vi "WOBOT 2020 Vision.vi"() -> ()   [LabVIEW 2025]
uses:
  Ctrls/Battery Control.ctl
  <vilib>/Utility/sysdir.llb/System Directory Type.ctl
  Camera Set Up/Event/Event Setup Types.ctl
  <vilib>/vision/Image Controls.llb/IMAQ Image.ctl
  <vilib>/Utility/config.llb/Read Key (String).vi
  <vilib>/Utility/config.llb/Write Key (String).vi
  <vilib>/Rock Robotics/Network Tables/NT Read Boolean.vi
  <vilib>/Rock Robotics/Network Tables/NT Read String.vi
  <vilib>/Rock Robotics/Network Tables/NT Write Boolean.vi
  <vilib>/Utility/config.llb/NI_LVConfig.lvlib
panel:
  in  "Tab Control":enum32{"Post Processed", "Post Processed 2"}(tab)
  in  "Exit":bool
  out "DS Talking":bool
  out "NT Table":bool
  out "Title":string="Wobot 2020 Vision Ver 1.0.6"
  in  "Save":bool
  out "Vision Computer IP Address":string="DESKTOP-BLQQPIQ"
  out "Attached Cameras":string[](array[string])
  out "Rio Talking":bool
  in  "TEAM":u32=141
  out "Vision Battery Power (%)":T1 scale=0.0..100.0
  out "Driver Station IP":string
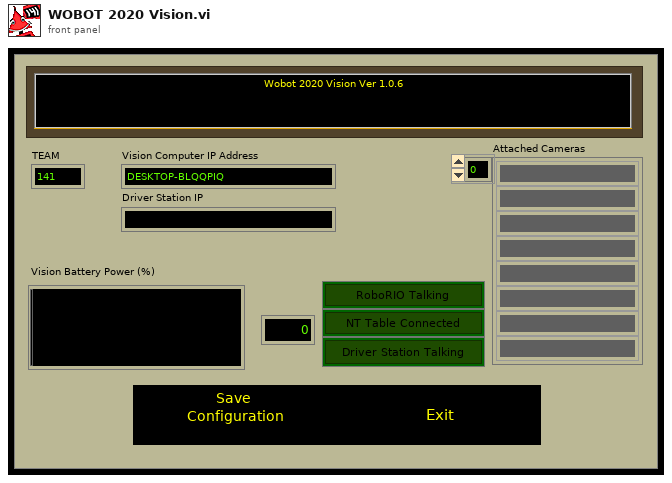
[diagram p1: front panel]
types:
  T1 = typedef "Battery Control.ctl" = u8
  T2 = typedef "System Directory Type.ctl" = i32
  T3 = typedef "Event Setup Types.ctl" = enum16{"Default", "Camera Loop Started", "GreyScale", "Reset Camera Settings", "Reset Team Number", "Save Data", "Setting Changed", "Update Video Mode", "Video Mode Changed", "Exit"}
  T4 = typedef "NI_LVConfig.lvlib/Config Data RefNum.ctl" = refnum<k1>
  T5 = typedef "IMAQ Image.ctl" = refnum<image>
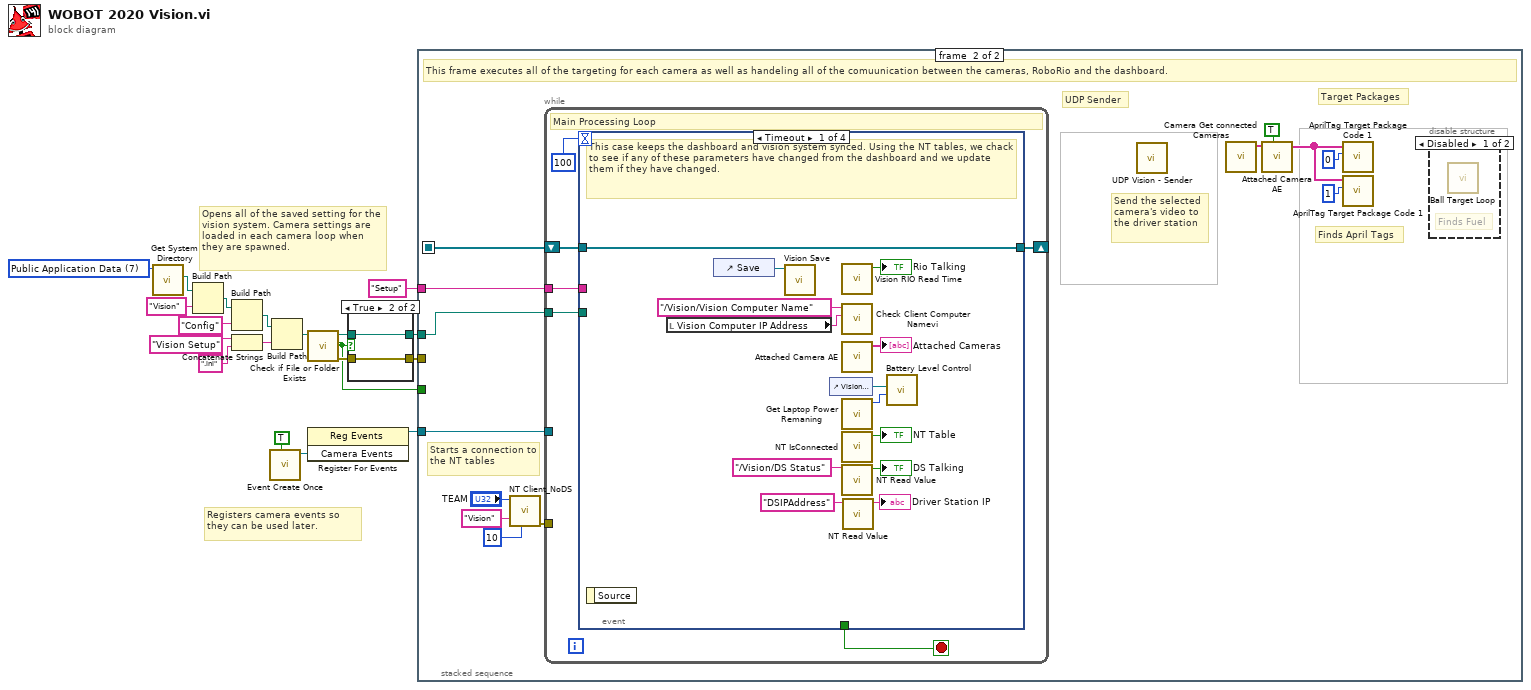
[diagram p0: block diagram]
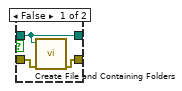
[diagram p2: hidden frame]
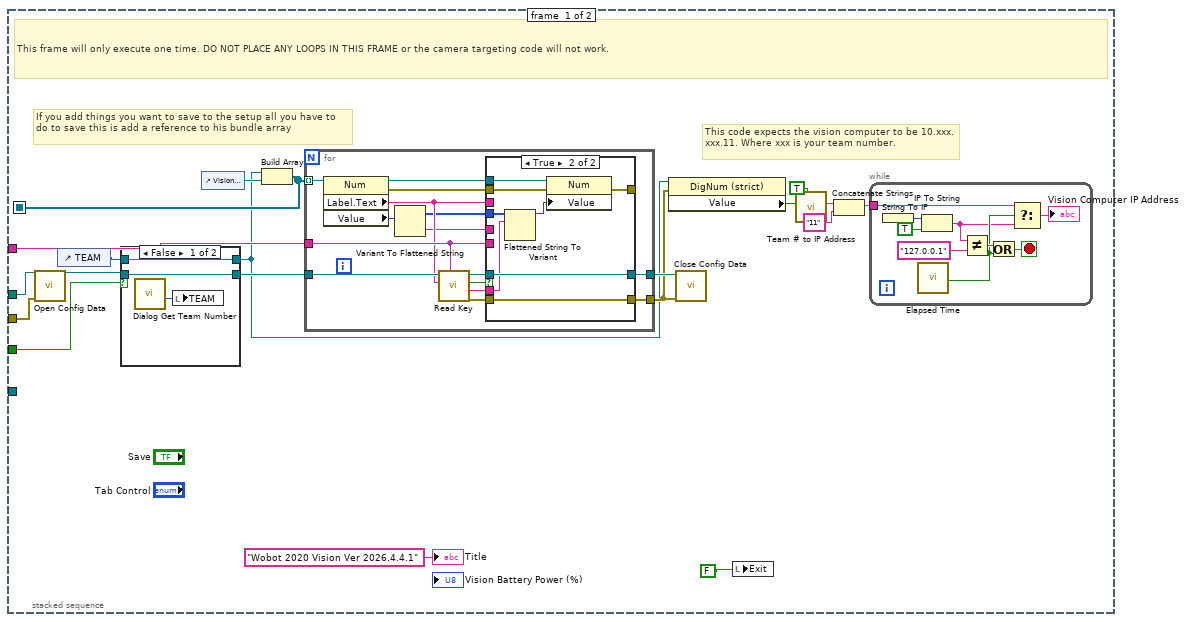
[diagram p3: hidden frame]
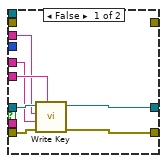
[diagram p4: hidden frame]
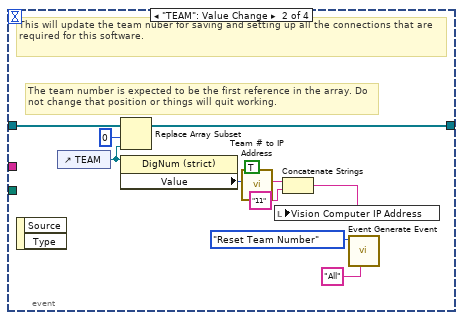
[diagram p7: hidden frame]
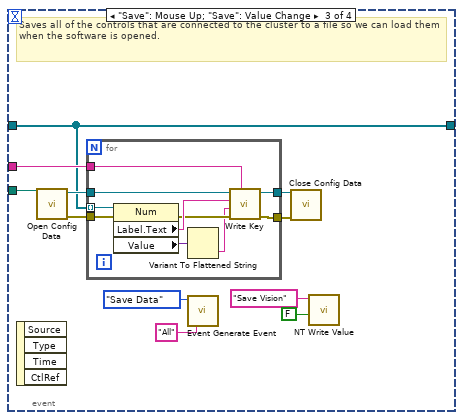
[diagram p8: hidden frame]
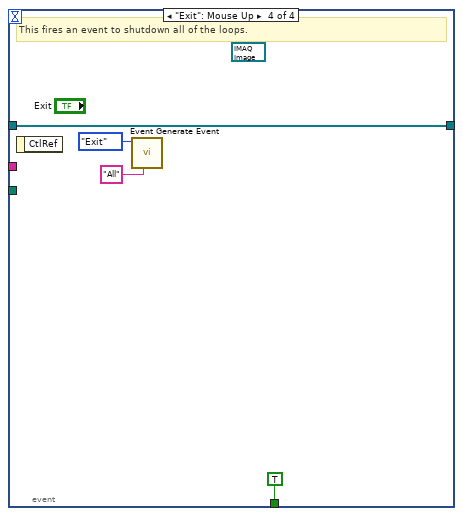
[diagram p9: hidden frame]
diagram:
  w4 = T2 7 items=["User Home"=0, "User Desktop"=1, "User Documents"=2, "User Application Data"=3, "User Preferences"=4, "User Temporary"=5, "Public Documents"=6, "Public Application Data"=7, "Public Preferences"=8, "Public Cache"=13, "System Core Libraries"=9, "System Installed Libraries"=10, "Application Files"=11, "Boot Volume Root"=12] ("system directory type")
  # "Opens all of the saved setting for the vision system. Camera settings are loaded in each camera loop when they are spawned."
  # "Registers camera events so they can be used later."
  n1 = call <vilib>:"Get System Directory.vi"("system directory type"=w4) -> ("system directory"=w3:path)  [unwired: 10 in]
  n2 = Build Path(base path=w3, name or relative path="Vision") -> (appended path=w1:path)
  n3 = Build Path(base path=w1, name or relative path="Config") -> (appended path=w11:path)
  n4 = Concatenate Strings("Vision Setup" ("name or relative path"), ".ini" ("name or relative path")) -> (w17:string)
  n5 = call "Event Create Once.vi"("ini"=TRUE) -> ("Camera Events"=w19:refnum<user-event>)  [unwired: 9 in, 1 out]
  n6 = Build Path(base path=w11, name or relative path=w17) -> (appended path=w12:path)
  n7 = call <vilib>:"Check if File or Folder Exists.vi"("path"=w12) -> ("error out"=w7:errorcluster, "file or folder exists?"=w5:bool, "dup path"=w9:path)  [unwired: 8 in]
  n8 = register-events(w19) -> (reference out=w18:refnum<event-registration>)  [unwired: 2 in, 1 out]
  n9 = case shown="True" w5 {
    tunnel: w9 -> [w22 w24]
    tunnel: [w22 w24] -> w8
    tunnel: w7 -> [w21 w23]
    tunnel: [w20 w23] -> w6
    frame False {
      n10 = call <vilib>:"Create File and Containing Folders.vi"("error in (no error)"=w21, "file path"=w22) -> ("error out"=w20:errorcluster)  [unwired: 8 in, 1 out]
    }
    frame True {
    }
  }
  n11 = stacked-sequence {
    seq-local: [w39 _] -> [_ w97]
    tunnel: w18 -> [_ w100]
    tunnel: w8 -> [w36 w99]
    tunnel: "Setup" ("Camera Name") -> [w38 w98]
    tunnel: w6 -> [w35 _]
    tunnel: w5 -> [w34 _]
    frame #0 {
      # "If you add things you want to save to the setup all you have to do to save this is add a reference to his bundle array"
      # "This code expects the vision computer to be 10.xxx.xxx.11. Where xxx is your team number."
      # "This frame will only execute one time. DO NOT PLACE ANY LOOPS IN THIS FRAME or the camera targeting code will not work."
      n12 = call <vilib>:"Open Config Data.vi"("error in (no error)"=w35, "configuration file path"=w36) -> ("refnum"=w37:T4)  [unwired: 7 in, 2 out]
      n13 = control-ref of="TEAM"() -> (w27:refnum<vi>)
      n14 = case shown="False" w34 {
        tunnel: w37 -> [w84 w87]
        tunnel: [w84 w87] -> w40
        tunnel: w27 -> [w83 w86]
        tunnel: [w83 w86] -> w26
        frame False {
          n15 = call "Dialog Get Team Number.vi"() -> ("Team Number"=w85:u32)  [unwired: 10 in]
          n16 = local write "TEAM"(w85) -> ()
        }
        frame True {
        }
      }
      n17 = control-ref of="Vision Battery Power (%)"() -> (w30:refnum<vi>)
      n18 = Build Array(w26, w30) -> (w39:refnum<vi>[])
      n19 = for {
        tunnel: w40 -> [w67]
        tunnel: w38 -> [w60]
        tunnel: w39 -> [w66] mode=indexing
        tunnel: [w58] -> w41
        tunnel: [w56] -> w33
        n20 = property class="Num"(reference=w66) -> (reference out=w63:refnum<vi>, error out=w62:errorcluster, "Label.Text"=w59:string, "Value"=w55:variant)  [unwired: 1 in]
        n21 = Variant To Flattened String(Variant=w55) -> (data string=w54:string, 1:w53:i16[])
        n22 = call-poly <vilib>:"Read Key.vi"("section"=w60, "key"=w59, "refnum"=w67) -> ("error out"=w57:errorcluster, "value"=w64:string, "found?"=w65:bool, "refnum out"=w61:T4)  [unwired: 5 in]
        n23 = case shown="True" w65 {
          tunnel: w64 -> [_ w77]
          tunnel: w63 -> [_ w82]
          tunnel: w62 -> [_ w81]
          tunnel: w61 -> [w74 w80]
          tunnel: w60 -> [w73 _]
          tunnel: w59 -> [w72 _]
          tunnel: [w71 w80] -> w58
          tunnel: w57 -> [w70 w79]
          tunnel: [w69 w79] -> w56
          tunnel: w54 -> [w68 _]
          tunnel: w53 -> [_ w78]
          tunnel: [_ w75] -> _
          frame False {
            n24 = call-poly <vilib>:"Write Key.vi"("section"=w73, "error in (no error)"=w70, "value"=w68, "key"=w72, "refnum"=w74) -> ("error out"=w69:errorcluster, "refnum out"=w71:T4)  [unwired: 4 in, 1 out]
          }
          frame True {
            n25 = Flattened String To Variant(6:w77, 7:w78) -> (3:w76:variant)  [unwired: 1 in, 1 out]
            n26 = property class="Num"(reference=w82, error in=w81, "Value"=w76) -> (error out=w75:errorcluster)  [unwired: 1 out]
          }
        }
      }
      n27 = property class="DigNum (strict)"(reference=w26, error in=w33) -> ("Value"=w32:u32)  [unwired: 2 out]
      n28 = call <vilib>:"Close Config Data.vi"("error in (no error)"=w33, "refnum"=w41) -> ()  [unwired: 8 in, 2 out]
      n29 = local write "Exit"(FALSE ("Exit")) -> ()
      n30 = call "Team # to IP Address.vi"("Update"=TRUE, "Team #"=w32) -> ("Team IP Address"=w31:string)  [unwired: 9 in]
      n31 = Concatenate Strings(w31, "11" ("string")) -> (w29:string)
      n32 = while {
        tunnel: w29 -> [w44]
        stop <- w48 stop-if-true
        n33 = String To IP() -> (0:w52:u32)  [unwired: 1 in]
        n34 = call "Elapsed Time"() -> ("Time has Elapsed"=w47:bool)  [unwired: 12 in, 7 out]
        n35 = IP To String(1:TRUE ("dot notation? (F)"), 2:w52) -> (0:w46:string)
        n36 = Not Equal?(x=w46, y="127.0.0.1") -> (x != y?=w49:bool)
        n37 = Or(x=w49, y=w47) -> (x .or. y?=w48:bool)
        n38 = Select(t=w44, s=w47, f=w46) -> (s? t:f=→"Vision Computer IP Address":string)
      }
      "Title" <- "Wobot 2020 Vision Ver 2026.4.4.1" ("Title")
    }
    frame #1 {
      # "Finds April Tags"
      # "UDP Sender"
      # "Target Packages"
      # "Send the selected camera's video to the driver station"
      # "Starts a connection to the NT tables"
      # "This frame executes all of the targeting for each camera as well as handeling all of the comuunication between the cameras, RoboRio and the dashboard."
      n39 = call "NT Client_NoDS.vi"("Update Time"=10, "Client Name"="Vision", "TEAM"="TEAM") -> ("error out"=w93:errorcluster)  [unwired: 8 in]
      n40 = while {
        tunnel: w100 -> [_]
        tunnel: w99 -> [w104]
        tunnel: w98 -> [w103]
        tunnel: w93 -> [_]
        shift-right: [w101] -> _
        shift-left: w97 -> [w102]
        stop <- w106 stop-if-true
        # "Main Processing Loop"
        n41 = event shown="[0] Timeout" {
          selector: _ -> [_ _ _ _]
          dyn-events: _ -> [_ _ _ _]
          timeout: 100 -> [_ _ _ _]
          tunnel: [_ _ _ TRUE] -> w106
          tunnel: w104 -> [_ _ w135 _]
          tunnel: w103 -> [_ _ w136 _]
          tunnel: w102 -> [w109 w130 w132 w153]
          tunnel: [w109 w128 w132 w153] -> w101
          event Timeout {
            # "This case keeps the dashboard and vision system synced. Using the NT tables, we chack to see if any of these parameters have changed from the dashboard and we update them if they have changed."
            n42 = event-data() -> ()  [unwired: 1 in, 1 out]
            n43 = local read "Vision Computer IP Address"() -> (w116:string)
            n44 = control-ref of="Save"() -> (w115:refnum<vi>)
            n45 = call "Vision Save.vi"("Save"=w115) -> ()  [unwired: 11 in]
            n46 = control-ref of="Vision Battery Power"() -> (w113:refnum<vi>)
            n47 = call "Vision RIO Read Time.vi"() -> ("Rio Talking"=→"Rio Talking":bool)  [unwired: 11 in]
            n48 = call "Check Client Computer Namevi.vi"("Computer DNS Name"=w116, "Name"="/Vision/Vision Computer Name") -> ()  [unwired: 10 in]
            n49 = call "Attached Camera AE.vi"() -> ("Camera List out"=→"Attached Cameras":string[])  [unwired: 11 in]
            n50 = call "Get Laptop Power Remaning.vi"() -> ("BatteryLifePercent"=w112:u8)  [unwired: 11 in]
            n51 = call "NT IsConnected.vi"() -> ("Connected"=→"NT Table":bool)  [unwired: 10 in, 1 out]
            n52 = call-poly <vilib>:"NT Read Value.vi"("name"="/Vision/DS Status" ("Name")) -> ("value"=→"DS Talking":bool)  [unwired: 8 in, 2 out]
            n53 = call-poly <vilib>:"NT Read Value.vi"("name"="DSIPAddress") -> ("value"=→"Driver Station IP":string)  [unwired: 8 in, 2 out]
            n54 = call "Battery Level Control.vi"("Power Level"=w112, "Battery Power ref"=w113) -> ()  [unwired: 10 in]
          }
          event "TEAM": Value Change {
            # "The team number is expected to be the first reference in the array. Do not change that position or things will quit working."
            # "This will update the team nuber for saving and setting up all the connections that are required for this software."
            n55 = event-data() -> ()  [unwired: 1 in, 2 out]
            n56 = control-ref of="TEAM"() -> (w125:refnum<vi>)
            n57 = Replace Array Subset(array=w130, new element=w125, index=0) -> (w128:refnum<vi>[])
            n58 = property class="DigNum (strict)"(reference=w125) -> ("Value"=w124:u32)  [unwired: 1 in, 2 out]
            n59 = call "Team # to IP Address.vi"("Update"=TRUE, "Team #"=w124) -> ("Team IP Address"=w127:string)  [unwired: 9 in]
            n60 = Concatenate Strings(w127, "11" ("string")) -> (w123:string)
            n61 = local write "Vision Computer IP Address"(w123) -> ()
            n62 = call "Event Generate Event.vi"("Camera Name"="All" ("y"), "Event Type"=Event_Setup_Types."Reset Team Number") -> ()  [unwired: 10 in]
          }
          event "Save": Mouse Up; "Save": Value Change {
            # "Saves all of the controls that are connected to the cluster to a file so we can load them when the software is opened."
            n63 = event-data() -> ()  [unwired: 1 in, 4 out]
            n64 = call <vilib>:"Open Config Data.vi"("configuration file path"=w135) -> ("error out"=w137:errorcluster, "refnum"=w140:T4)  [unwired: 8 in, 1 out]
            n65 = for {
              tunnel: w132 -> [w149] mode=indexing
              tunnel: w140 -> [w151]
              tunnel: w136 -> [w150]
              tunnel: [w146] -> w139
              tunnel: [w144] -> w138
              tunnel: w137 -> [w143]
              n66 = property class="Num"(reference=w149, error in=w143) -> (error out=w145:errorcluster, "Label.Text"=w148:string, "Value"=w147:variant)  [unwired: 1 out]
              n67 = Variant To Flattened String(Variant=w147) -> (data string=w142:string)  [unwired: 1 out]
              n68 = call-poly <vilib>:"Write Key.vi"("section"=w150, "error in (no error)"=w145, "value"=w142, "key"=w148, "refnum"=w151) -> ("error out"=w144:errorcluster, "refnum out"=w146:T4)  [unwired: 4 in, 1 out]
            }
            n69 = call "Event Generate Event.vi"("Camera Name"="All" ("y"), "Event Type"=Event_Setup_Types."Save Data") -> ()  [unwired: 10 in]
            n70 = call <vilib>:"Close Config Data.vi"("error in (no error)"=w138, "refnum"=w139) -> ()  [unwired: 8 in, 2 out]
            n71 = call-poly <vilib>:"NT Write Value.vi"("value"=FALSE ("Boolean"), "name"="Save Vision" ("Name")) -> ()  [unwired: 9 in, 1 out]
          }
          event "Exit": Mouse Up {
            (unwired) T5 refnum ("Image")
            # "This fires an event to shutdown all of the loops."
            n72 = event-data() -> ()  [unwired: 1 in, 1 out]
            n73 = call "Event Generate Event.vi"("Camera Name"="All" ("y"), "Event Type"=Event_Setup_Types."Exit") -> ()  [unwired: 10 in]
          }
        }
      }
      n74 = call "UDP Vision - Sender.vi"() -> ()  [unwired: 12 in]
      n75 = call "Camera Get connected Cameras.vi"() -> ("Camera List"=w92:string[])  [unwired: 10 in, 1 out]
      n76 = call "Attached Camera AE.vi"("Update"=TRUE, "Camera List in"=w92) -> ("Camera List out"=w90:string[])  [unwired: 9 in]
      n77 = call "AprilTag Target Package Code 1.vi"("Camera List"=w90, "Instance"=0) -> ()  [unwired: 9 in]
      n78 = call "AprilTag Target Package Code 1.vi"("Camera List"=w90, "Instance"=1) -> ()  [unwired: 9 in]
      n79 = disable-structure shown="Disabled" {
        frame Disabled {
          # "Finds Fuel"
          n80 = call "Ball Target Loop.vi"() -> ()  [unwired: 11 in]
        }
        frame Enabled {
        }
      }
    }
  }
